vi "implementation_node.vi"() -> ()   [LabVIEW 2018]
uses:
  <vilib>/Utility/xml.llb/Read From XML File(string).vi
panel:
  in  "Data file":path
  out "Output":dbl
  in  "Weights XML\n(Select Existing File)":path
  # "Neural Network Implementation Node"
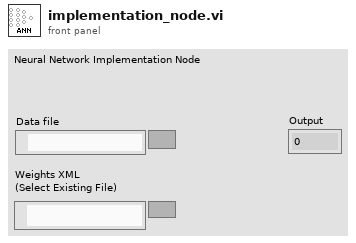
[diagram p1: front panel]
types:
  T1 = cluster{cluster{dbl[][], dbl[][], dbl[][]}, cluster{dbl[], dbl[], dbl[]}}
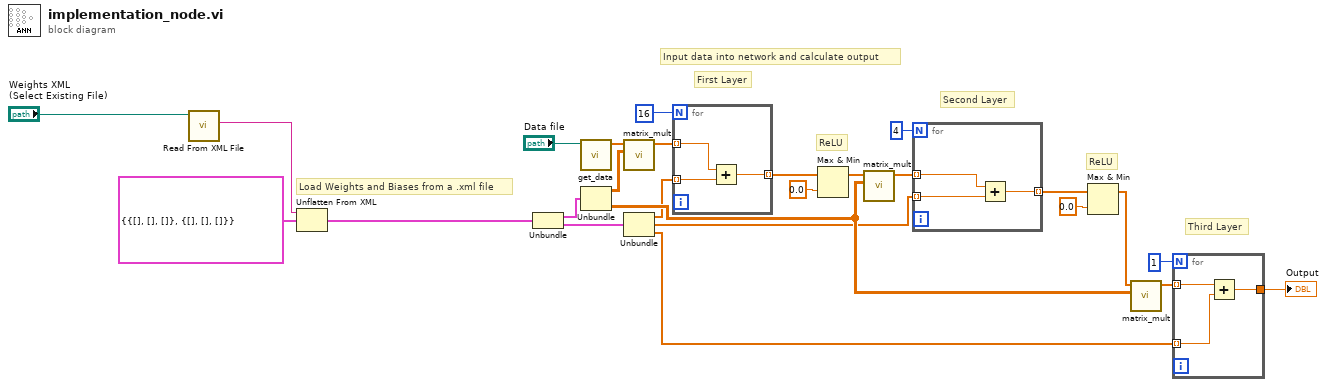
[diagram p0: block diagram]
diagram:
  # "Third Layer"
  # "Second Layer"
  # "First Layer"
  # "ReLU"
  # "ReLU"
  # "Load Weights and Biases from a .xml file"
  # "Input data into network and calculate output"
  n1 = call-poly <vilib>:"Read From XML File.vi"("XML File Path"="Weights XML\n(Select Existing File)") -> ("XML Elements"=w24:string)  [unwired: 8 in, 2 out]
  n2 = Unflatten From XML(xml string=w24, type=T1 {{[], [], []}, {[], [], []}}) -> (value=w25:T1)  [unwired: 1 in, 1 out]
  n3 = Unbundle(w25) -> (w6:cluster{dbl[][], dbl[][], dbl[][]}, w5:cluster{dbl[], dbl[], dbl[]})
  n4 = call "get_data.vi"("file (use dialog)"="Data file") -> ("Raw Data"=w1:dbl[])  [unwired: 9 in, 1 out]
  n5 = Unbundle(w6) -> (w14:dbl[][], w13:dbl[][])  [unwired: 1 out]
  n6 = call "matrix_mult.vi"("Weights"=w14, "Input Array"=w1) -> ("Matrix Product"=w4:dbl[])  [unwired: 9 in]
  n7 = Unbundle(w5) -> (w12:dbl[], w11:dbl[], w10:dbl[])
  n8 = for {
    N: 16 -> [_]
    tunnel: [w29] -> w22 mode=indexing
    tunnel: w4 -> [w28] mode=indexing
    tunnel: w12 -> [w27] mode=indexing
    n9 = Add(x=w28, y=w27) -> (x+y=w29:dbl)
  }
  n10 = Max & Min(x=w22, y=0.0) -> (max(x,y)=w9:dbl[])  [unwired: 1 out]
  n11 = call "matrix_mult.vi"("Weights"=w13, "Input Array"=w9) -> ("Matrix Product"=w8:dbl[])  [unwired: 9 in]
  n12 = for {
    N: 4 -> [_]
    tunnel: [w32] -> w16 mode=indexing
    tunnel: w8 -> [w31] mode=indexing
    tunnel: w11 -> [w30] mode=indexing
    n13 = Add(x=w31, y=w30) -> (x+y=w32:dbl)
  }
  n14 = Max & Min(x=w16, y=0.0) -> (max(x,y)=w7:dbl[])  [unwired: 1 out]
  n15 = call "matrix_mult.vi"("Weights"=w13, "Input Array"=w7) -> ("Matrix Product"=w15:dbl[])  [unwired: 9 in]
  n16 = for {
    N: 1 -> [_]
    tunnel: [w35] -> w3
    tunnel: w15 -> [w34] mode=indexing
    tunnel: w10 -> [w33] mode=indexing
    n17 = Add(x=w34, y=w33) -> (x+y=w35:dbl)
  }
  "Output" <- w3
